vi "Tusk.Kill.vi"(8 "error in (no error)":errorcluster, 9 "Data":variant, 11 "Tusk in":refnum<class "Tusk.lvclass">) -> (0 "error out":errorcluster, 3 "Tusk out":refnum<class "Tusk.lvclass">)   [LabVIEW 2018, in "Application.lvlib" / "Tusk.lvclass"]
uses:
  Tusk.lvclass
  Tusk.lvclass/Tusk.ctl
  Message Class/Message.lvclass/Message.ctl
  Exceptions Class/VIs/Invalid Type.vi
  <vilib>/Utility/error.llb/Trim Whitespace.vi
  Message Class/Message.lvclass
  Keywords Class/Keywords.lvclass
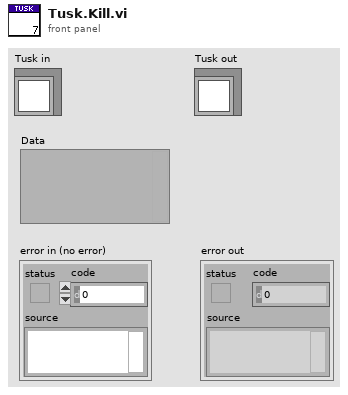
[diagram p1: front panel]
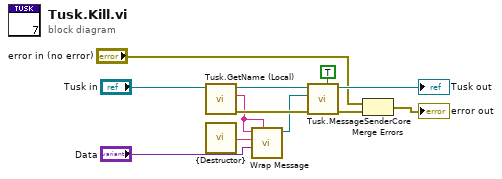
[diagram p0: block diagram]
diagram:
  n1 = call "Tusk.GetName (Local).vi"("Tusk in"="Tusk in") -> ("error out"=w12:errorcluster, "Name(Local)"=w7:string, "Tusk out"=w6:refnum<class "Tusk.lvclass">)  [unwired: 8 in]
  n2 = call "{Destructor}.vi"() -> ("Word"=w4:string)  [unwired: 6 in]
  n3 = call "Wrap Message.vi"("Sender"=w7, "Data"="Data", "Message"=w4, "Recipient"=w7) -> ("Message out"=w5:refnum<class "Message.lvclass">)  [unwired: 6 in, 1 out]
  n4 = call "Tusk.MessageSenderCore.vi"("Priority?"=TRUE, "error in (no error)"=w12, "Message"=w5, "Tusk in"=w6) -> ("error out"=w11:errorcluster, "Tusk out"=→"Tusk out":refnum<class "Tusk.lvclass">)  [unwired: 5 in, 1 out]
  n5 = Merge Errors("error in (no error)", w11) -> (→"error out":errorcluster)
